vi "HTTPRPC_delete.vi"(0 "mbed_LVLibrary.lvlib:mbed.lvclass":refnum<class "mbed.lvclass">, 3 "error in (no error)":errorcluster) -> (10 "error out":errorcluster)   [LabVIEW 2011, in "mbed_LVLibrary.lvlib" / "HTTPRPC.lvclass"]
uses:
  HTTPRPC.lvclass
  mbed/mbed.lvclass
panel:
  in  "mbed_LVLibrary.lvlib:HTTPRPC.lvclass":refnum<class "HTTPRPC.lvclass">
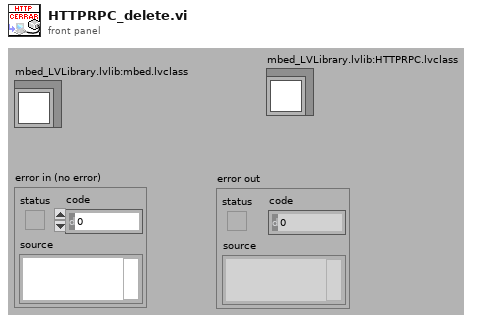
[diagram p1: front panel]
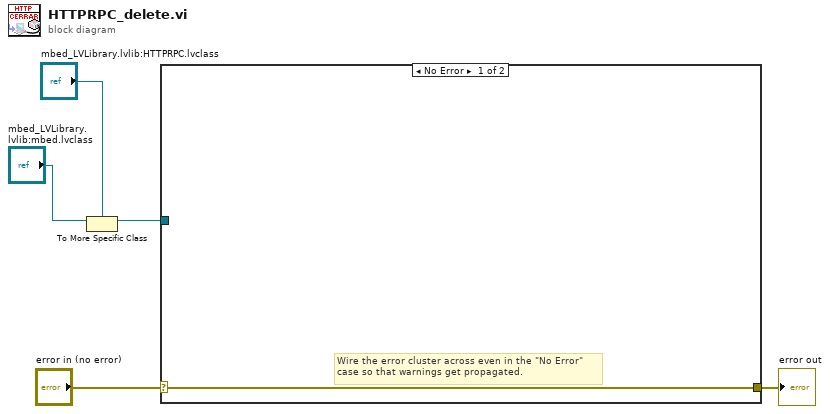
[diagram p0: block diagram]
diagram:
  n1 = To More Specific Class(target class="mbed_LVLibrary.lvlib:HTTPRPC.lvclass", reference="mbed_LVLibrary.lvlib:mbed.lvclass") -> (specific class reference=w2:refnum<class "HTTPRPC.lvclass">)  [unwired: 1 in, 1 out]
  n2 = case shown="No Error" "error in (no error)" {
    selector: "error in (no error)" -> [w6 w7]
    tunnel: [w6 w7] -> w4
    tunnel: w2 -> [_ _]
    frame No Error {
      # "Wire the error cluster across even in the \"No Error\"\ncase so that warnings get propagated."
    }
    frame Error {
    }
  }
  "error out" <- w4
